vi "PH_Revolver-GUI_6P.constructor.vi"(0 "name":string, 2 "data in":string, 5 "error in(no error)":errorcluster) -> (14 "i ref out":refnum<vi>, 16 "data out":string, 19 "error out":errorcluster)   [LabVIEW 2014, in "PH_Revolver-GUI_6P.lvlib"]
doc: "This class is forseen to control up to two Sixpack Axes (classes: Trinamic_Axis and Trinamic_Controller).\n\nThis class is part of the PHELIX user layer.\n\nauthor: Stefan Götte, GSI\n\nLicense Agreement for this software:\n\nCopyright (C)\nGesellschaft für Schwerionenforschung, GSI\nPlanckstr. 1\n64291 Darmstadt\nGermany\n\nContact: D.Beck@gsi.de \n\nThis program is free software; you can redistribute it and/or modify it under the terms of the \nGNU General Public License as published by the Free Software Foundation; either version 2 of \nthe license, or (at your option) any later version.\n\nThis program is distributed in the hope that it will be useful, but WITHOUT ANY WARRANTY; \nwithout even the implied warranty of MERCHANTABILITY or FITNESS FOR A PARTICULAR PURPOSE. See the GNU General License for more details (http://www.gnu.org).\n\nGesellschaft für Schwerionenforschung, GSI\nPlanckstr. 1, 64291 Darmstadt, Germany\nFor all questions and ideas contact: M.Richter@gsi.de, H.Brand@gsi.de or D.Beck@gsi.de.\nLast update: 16-JUN-2004"
uses:
  PH_Revolver-GUI_6P.lvlib
  CS_Core/CSObj/CSObj.lvlib
  PH_Basics/PH_AxisGUI_BaseClass/PH_AxisGUI_BaseClass.lvlib
  PH_Basics/PH_Class/PH_Class.lvlib
  PH_Basics/PH_PSDBWriter/PH_PSDBWriter.lvlib
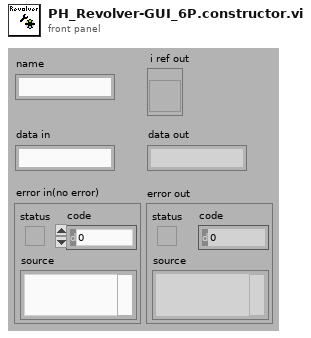
[diagram p1: front panel]
types:
  T1 = enum16{"SetAttribute", "GetAttribute", "CreateAttribute", "DestroyAttribute", "DestroyAllAtributes"}
  T2 = typedef "PH_Revolver-GUI_6P.lvlib/PH_Revolver-GUI_6P.i attribute.ctl" = cluster{"GUI Refs":cluster{"0°":refnum<vi>, "60°":refnum<vi>, "120°":refnum<vi>, "180°":refnum<vi>, "240°":refnum<vi>, "300°":refnum<vi>, "Action":refnum<vi>}, "Revolver Position":T3, "Service ID Position":i32, "Captions":string[]}
  T3 = typedef "PH_Revolver-GUI_6P.lvlib/PH_Revolver-GUI_6P.Position.ctl" = u16
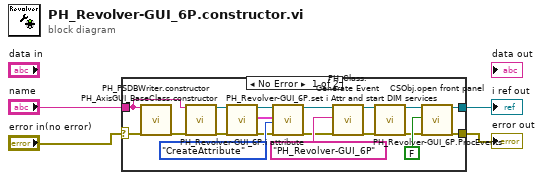
[diagram p0: block diagram]
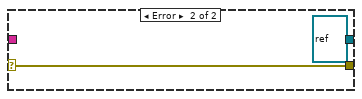
[diagram p2: hidden frame]
diagram:
  n1 = case shown="No Error" "error in(no error)" {
    selector: "error in(no error)" -> [w22 w25]
    tunnel: [w20 w25] -> w4
    tunnel: [w21 refnum<vi> refnum ("i ref out")] -> w3
    tunnel: "name" -> [w19 _]
    frame No Error {
      n2 = call "PH_PSDBWriter.constructor.vi"("name"=w19, "error in"=w22) -> ("error out"=w10:errorcluster)  [unwired: 15 in, 2 out]
      n3 = call "PH_AxisGUI_BaseClass.constructor.vi"("name"=w19, "error in(no error)"=w10) -> ("i ref out"=w9:refnum<vi>, "error out"=w7:errorcluster)  [unwired: 15 in, 1 out]
      n4 = call "PH_Revolver-GUI_6P.set i Attr and start DIM services.vi"("i ref in"=w9, "error in (no error)"=w7) -> ("i ref out"=w8:refnum<vi>, "i Attributes"=w5:T2, "error out"=w6:errorcluster)  [unwired: 15 in]
      n5 = call "PH_Revolver-GUI_6P.i attribute.vi"("VI Refnum"=w8, "CLASS.i attribute"=w5, "Action"=T1."CreateAttribute", "error in (no error)"=w6) -> ("VI Refnum out"=w12:refnum<vi>, "error out"=w14:errorcluster)  [unwired: 13 in, 1 out]
      n6 = call "PH_Class.Generate Event.vi"("i ref in"=w12, "Class"="PH_Revolver-GUI_6P", "error in (no error)"=w14) -> ("i ref out"=w11:refnum<vi>, "error out"=w13:errorcluster)  [unwired: 15 in]
      n7 = call "PH_Revolver-GUI_6P.ProcEvents.vi"("i ref in"=w11, "error in"=w13) -> ("i ref out"=w16:refnum<vi>, "error out"=w15:errorcluster)  [unwired: 16 in]
      n8 = call "CSObj.open front panel.vi"("i ref in"=w16, "frontPanelOpen"=FALSE ("front panel open"), "error in (no error)"=w15) -> ("i ref out"=w21:refnum<vi>, "error out"=w20:errorcluster)  [unwired: 15 in]
    }
    frame Error {
    }
  }
  "i ref out" <- w3
  "error out" <- w4
